vi "format_offset_config.vi"(11 "config":T2={"mag.o"={"x"=0.0, "y"=0.0, "z"=0.0}, "mag.r"=1.0, "acc.o"={"x"=0.0, "y"=0.0, "z"=0.0}, "acc.r"=1.0, "gyr.o"={"x"=0.0, "y"=0.0, "z"=0.0}}) -> (3 "initial config":string="#define OFFSET_MAG_X 0.00\n#define OFFSET_MAG_Y 0.00\n#define OFFSET_MAG_Z 0.00\n#define R_MAG 1.00\n\n#define OFFSET_ACC_X 0.00\n#define OFFSET_ACC_Y 0.00\n#define OFFSET_ACC_Z 0.00\n#define R_ACC 1.00\n\n#define OFFSET_GYR_X 0.00\n#define OFFSET_GYR_Y 0.00\n#define OFFSET_GYR_Z 0.00")   [LabVIEW 2019, in "Nano33BLE-TiltCompensationSupport.lvlib"]
uses:
  types/xyz.ctl
  Nano33BLE-TiltCompensationSupport.lvlib
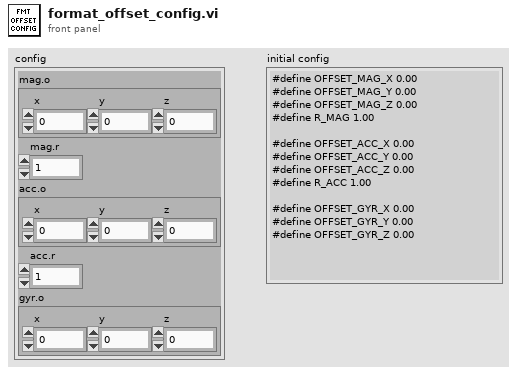
[diagram p1: front panel]
types:
  T1 = typedef "Nano33BLE-TiltCompensationSupport.lvlib/xyz.ctl" = cluster{"x":dbl, "y":dbl, "z":dbl}
  T2 = cluster{"mag.o":T1, "mag.r":dbl, "acc.o":T1, "acc.r":dbl, "gyr.o":T1}
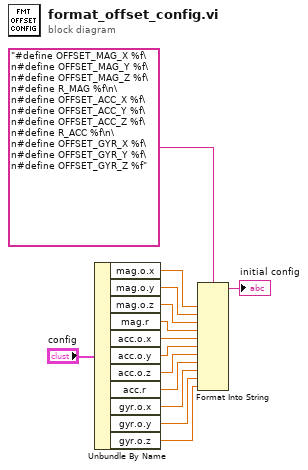
[diagram p0: block diagram]
diagram:
  n1 = Unbundle By Name("config") -> ("mag.o.x"=w11:dbl, "mag.o.y"=w10:dbl, "mag.o.z"=w9:dbl, "mag.r"=w8:dbl, "acc.o.x"=w7:dbl, "acc.o.y"=w6:dbl, "acc.o.z"=w5:dbl, "acc.r"=w4:dbl, "gyr.o.x"=w3:dbl, "gyr.o.y"=w2:dbl, "gyr.o.z"=w1:dbl)
  n2 = Format Into String(format string="#define OFFSET_MAG_X %f\n#define OFFSET_MAG_Y %f\n#define OFFSET_MAG_Z %f\n#define R_MAG %f\n\n#define OFFSET_ACC_X %f\n#define OFFSET_ACC_Y %f\n#define OFFSET_ACC_Z %f\n#define R_ACC %f\n\n#define OFFSET_GYR_X %f\n#define OFFSET_GYR_Y %f\n#define OFFSET_GYR_Z %f", w11, w10, w9, w8, w7, w6, w5, w4, w3, w2, w1) -> (resulting string=→"initial config":string)  [unwired: 2 in, 1 out]
